vi "Main.vi"(11 "Module Admin":refnum<class "Delacor_lib_QMH_Module Admin.lvclass">) -> ()   [LabVIEW 2019, in "UI.lvlib"]
doc: "This template is based off of the Queued Message Handler design pattern and the Queued Message Handler project template that ships with LabVIEW.\n\nThe main difference is that the queue is private to this module and communication between modules is performed via Broadcast and Request events.\n\nRequest events are wrapped in public API methods and are handled in the Event Handling Loop (EHL) of this VI. Any module can register for Broadcast events sent by this module. The EHL generates messages based on user interface actions.\n\nThe Message Handling Loop (MHL) processes messages generated by the EHL, or by other messages. The messages are string values, so new messages can be added easily to the Message Cases case structure in the MHL. Each message cluster can also provide an optional value for Message Data, which is a variant that can be converted to whatever message-specific data is required.\n_____\nBased on Delacor QMH Project Template 5.0.0.82."
uses:
  UI.lvlib
  <vilib>/Delacor/Delacor QMH/Libraries/Module Admin_class/Delacor_lib_QMH_Module Admin.lvclass
  Module Data--cluster.ctl
  Stop Argument--cluster.ctl
  <vilib>/Delacor/Delacor QMH/Libraries/Message Queue_class/Delacor_lib_QMH_Message Queue.lvclass/Delacor_lib_QMH_Message Queue.ctl
  <vilib>/Delacor/Delacor QMH/Libraries/Module Admin_class/Delacor_lib_QMH_Module Admin.lvclass/Delacor_lib_QMH_Module Admin.ctl
  <vilib>/Delacor/Delacor QMH/Libraries/Message Queue_class/Delacor_lib_QMH_Enqueue Message (Single).vi
  <vilib>/Delacor/Delacor QMH/Libraries/Module Admin_class/Delacor_lib_QMH_Get External Launch.vi
  <vilib>/Utility/error.llb/Error Cluster From Error Code.vi
  <vilib>/ErrorRing/Error Ring.xnode
  <vilib>/Delacor/Delacor QMH/Libraries/Message Queue_class/Delacor_lib_QMH_Message Queue.lvclass
  Analisis/Analisis.lvlib
  Mensajes/Mensajes.lvlib
  Configuracion/Configuracion.lvlib
  Adquisicion_Helper_Loop/Adquisicion_Helper_Loop.lvlib
  Save DB_SQLite/Save DB_SQLite.lvlib
panel:
  out "error out":errorcluster
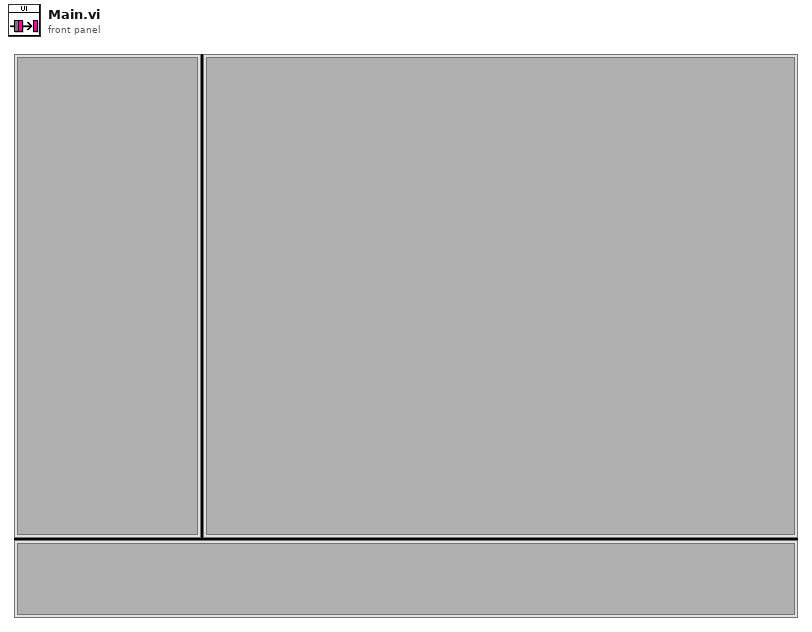
[diagram p1: front panel]
types:
  T1 = typedef "UI.lvlib/Request Events--cluster.ctl" = cluster{"Stop Module":refnum<user-event>, "Show Panel":refnum<user-event>, "Hide Panel":refnum<user-event>, "Get Module Execution Status":refnum<user-event>, "Show Diagram":refnum<user-event>}
  T2 = typedef "Configuracion.lvlib/Broadcast Events--cluster.ctl" = cluster{"Module Did Init":refnum<user-event>, "Status Updated":refnum<user-event>, "Error Reported":refnum<user-event>, "Module Did Stop":refnum<user-event>, "Update Module Execution Status":refnum<user-event>}
  T3 = typedef "Save DB_SQLite.lvlib/Broadcast Events--cluster.ctl" = cluster{"Module Did Init":refnum<user-event>, "Status Updated":refnum<user-event>, "Error Reported":refnum<user-event>, "Module Did Stop":refnum<user-event>, "Update Module Execution Status":refnum<user-event>}
  T4 = typedef "Mensajes.lvlib/Broadcast Events--cluster.ctl" = cluster{"Module Did Init":refnum<user-event>, "Status Updated":refnum<user-event>, "Error Reported":refnum<user-event>, "Module Did Stop":refnum<user-event>, "Update Module Execution Status":refnum<user-event>}
  T5 = typedef "Adquisicion_Helper_Loop.lvlib/Broadcast Events--cluster.ctl" = cluster{"Module Did Init":refnum<user-event>, "Status Updated":refnum<user-event>, "Error Reported":refnum<user-event>, "Module Did Stop":refnum<user-event>, "Update Module Execution Status":refnum<user-event>}
  T6 = typedef "Analisis.lvlib/Broadcast Events--cluster.ctl" = cluster{"Module Did Init":refnum<user-event>, "Status Updated":refnum<user-event>, "Error Reported":refnum<user-event>, "Module Did Stop":refnum<user-event>, "Update Module Execution Status":refnum<user-event>}
  T7 = typedef "UI.lvlib/Module Data--cluster.ctl" = cluster{"Status":string}
  T8 = enum32{"invalid lock state", "Not Locked", "Locked (No Password)", "Password-protected"}
  T9 = typedef "UI.lvlib/Stop Argument--cluster.ctl" = cluster{"Origin":string, "Exit via Stop Module Req?":bool, "Wait for Module to stop?":bool}
  T10 = enum32{"Invalid", "Standard", "Closed", "Hidden", "Minimized", "Maximized"}
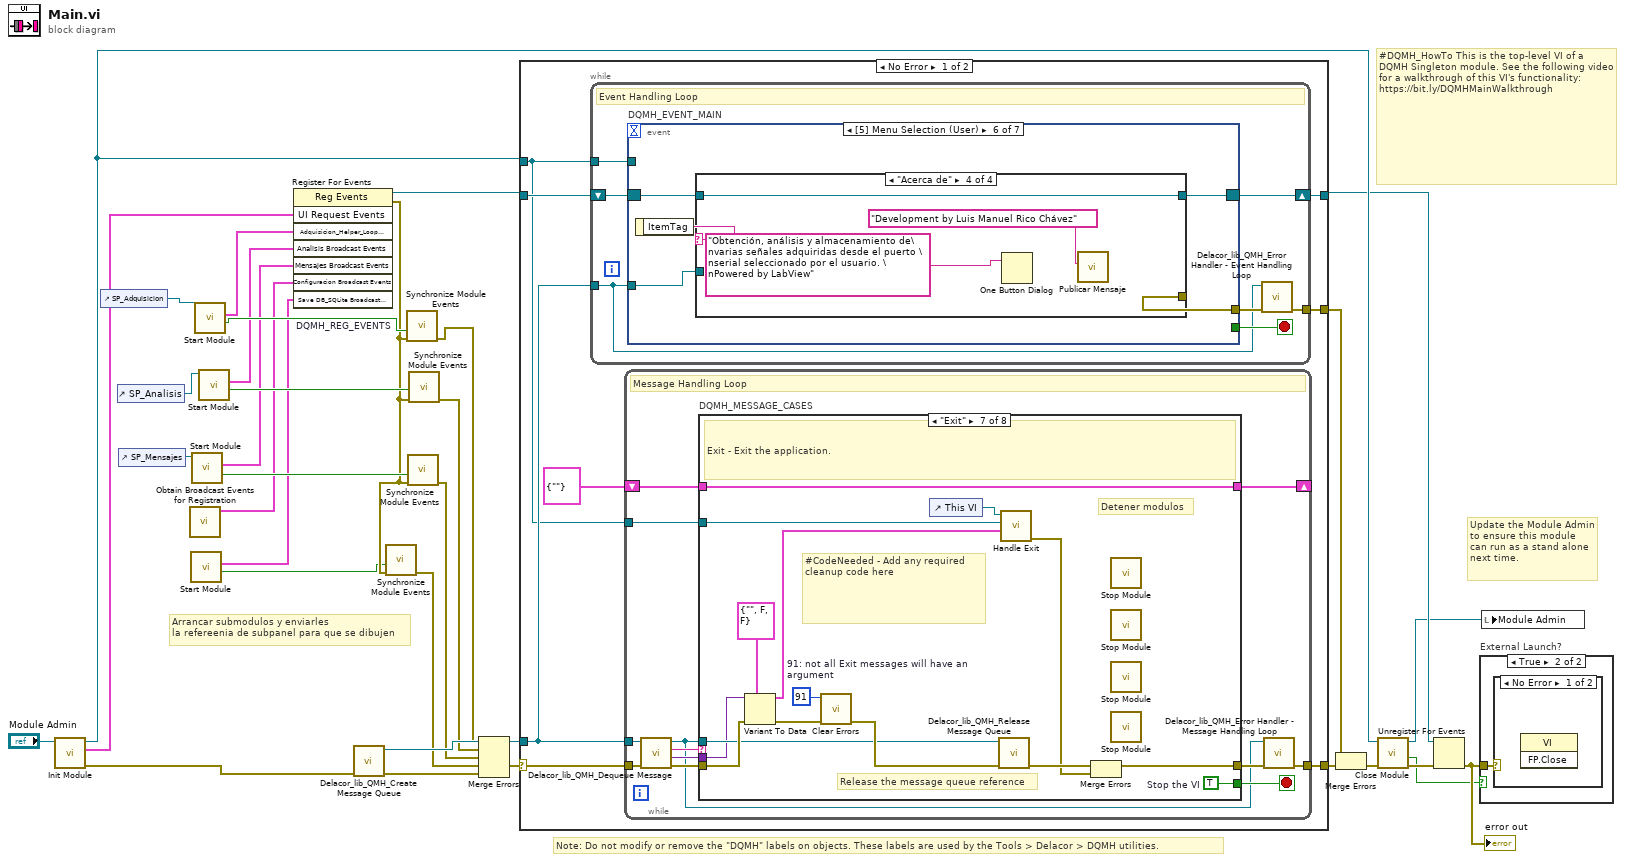
[diagram p0: block diagram]
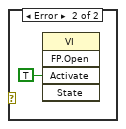
[diagram p3: hidden frame]
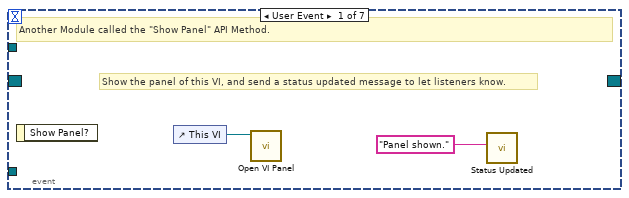
[diagram p4: hidden frame]
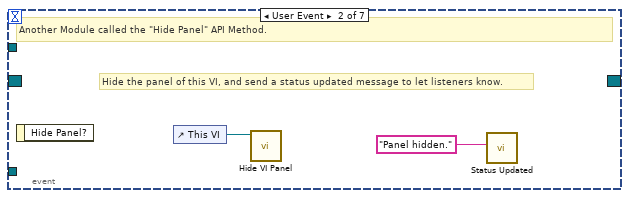
[diagram p5: hidden frame]
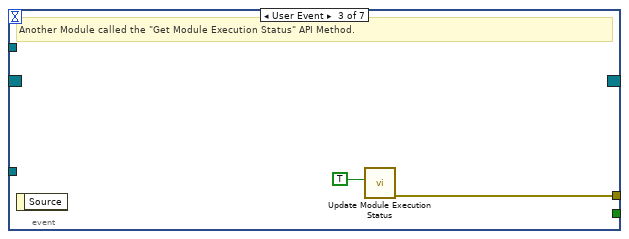
[diagram p6: hidden frame]
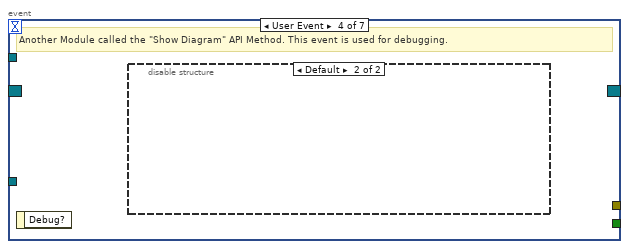
[diagram p7: hidden frame]
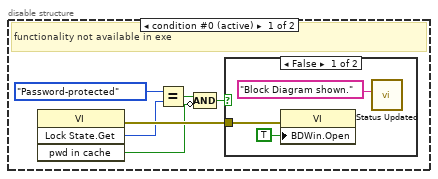
[diagram p8: hidden frame]
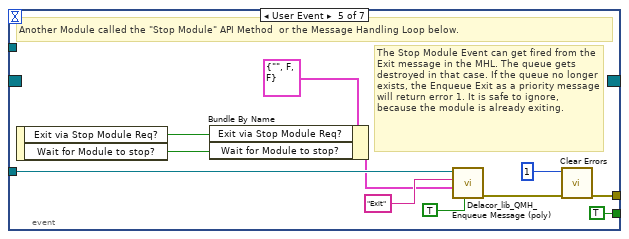
[diagram p10: hidden frame]
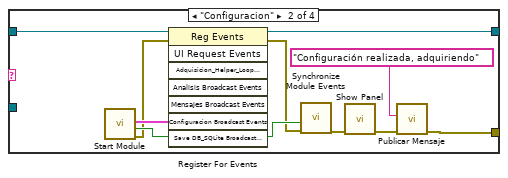
[diagram p12: hidden frame]
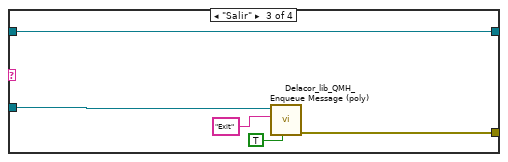
[diagram p13: hidden frame]
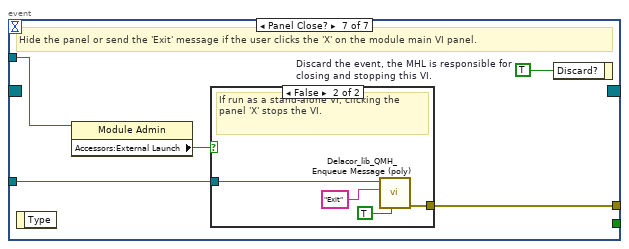
[diagram p14: hidden frame]
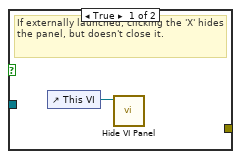
[diagram p15: hidden frame]
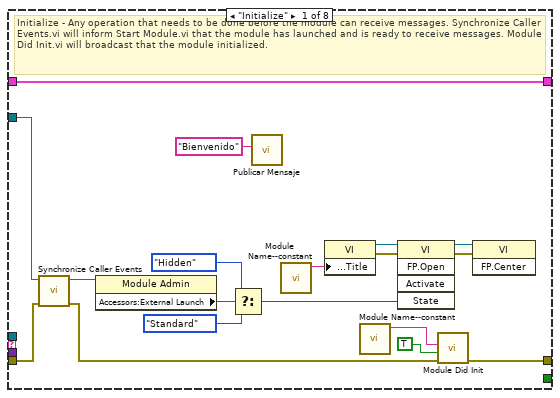
[diagram p16: hidden frame]
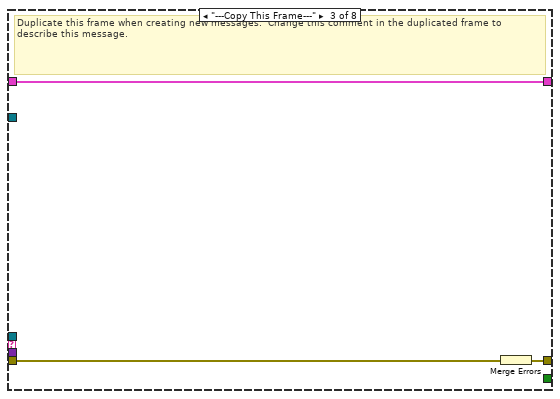
[diagram p18: hidden frame]
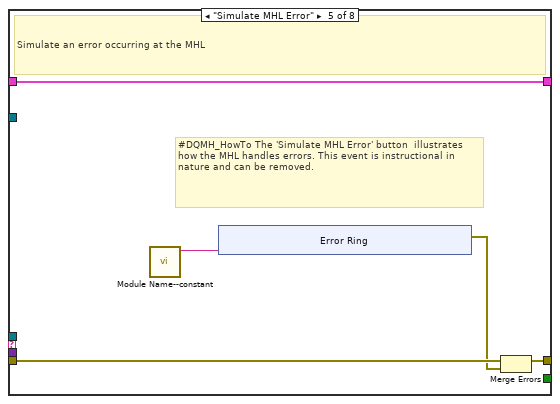
[diagram p20: hidden frame]
diagram:
  # "Arrancar submodulos y enviarles\nla refereenia de subpanel para que se dibujen"
  # "#DQMH_HowTo This is the top-level VI of a DQMH Singleton module. See the following video for a walkthrough of this VI's functionality: https://bit.ly/DQMHMainWalkthrough"
  # "Note: Do not modify or remove the \"DQMH\" labels on objects. These labels are used by the Tools > Delacor > DQMH utilities."
  # "Update the Module Admin to ensure this module can run as a stand alone next time."
  n1 = call "Init Module.vi"("Singleton Module Admin in"="Module Admin") -> ("error out"=w32:errorcluster, "UI Request Events"=w23:T1, "Singleton Module Admin out"=w26:refnum<class "Delacor_lib_QMH_Module Admin.lvclass">)  [unwired: 8 in]
  n2 = control-ref of="SP_Adquisicion"() -> (w9:refnum<vi>)
  n3 = control-ref of="SP_Analisis"() -> (w8:refnum<vi>)
  n4 = control-ref of="SP_Mensajes"() -> (w7:refnum<vi>)
  n5 = call "Obtain Broadcast Events for Registration.vi"() -> ("Configuracion Broadcast Events"=w6:T2)  [unwired: 9 in, 2 out]
  n6 = call "Start Module.vi"() -> ("Wait for Event Sync?"=w1:bool, "Save DB_SQLite Broadcast Events"=w5:T3)  [unwired: 8 in, 2 out]
  n7 = call "Start Module.vi"("SP_Mensajes"=w7) -> ("Wait for Event Sync?"=w16:bool, "Mensajes Broadcast Events"=w10:T4)  [unwired: 7 in, 2 out]
  n8 = call "Start Module.vi"("Sub Panel"=w9) -> ("Wait for Event Sync?"=w18:bool, "Adquisicion_Helper_Loop Broadcast Events"=w12:T5)  [unwired: 7 in, 2 out]
  n9 = call "Start Module.vi"("SP_Analisis"=w8) -> ("Wait for Event Sync?"=w17:bool, "Analisis Broadcast Events"=w11:T6)  [unwired: 7 in, 2 out]
  n10 = register-events "DQMH_REG_EVENTS"(w23, w12, w11, w10, w6, w5) -> (reference out=w24:refnum<event-registration>, error out=w2:errorcluster)  [unwired: 2 in]
  n11 = call <vilib>:"Delacor_lib_QMH_Create Message Queue.vi"("error in (no error)"=w32) -> ("error out"=w4:errorcluster, "Message Queue"=w22:refnum<class "Delacor_lib_QMH_Message Queue.lvclass">)  [unwired: 9 in]
  n12 = call "Synchronize Module Events.vi"("error in (no error)"=w2, "Wait for Event Sync?"=w1) -> ("error out"=w3:errorcluster)  [unwired: 9 in]
  n13 = call "Synchronize Module Events.vi"("error in (no error)"=w2, "Wait for Event Sync?"=w18) -> ("error out"=w13:errorcluster)  [unwired: 9 in]
  n14 = call "Synchronize Module Events.vi"("error in (no error)"=w2, "Wait for Event Sync?"=w16) -> ("error out"=w15:errorcluster)  [unwired: 9 in]
  n15 = call "Synchronize Module Events.vi"("error in (no error)"=w2, "Wait for Event Sync?"=w17) -> ("error out"=w14:errorcluster)  [unwired: 9 in]
  n16 = Merge Errors(w13, w14, w15, w3, w4) -> (w27:errorcluster)
  n17 = case shown="No Error" w27 {
    selector: w27 -> [w39 w206]
    tunnel: [w41 w205] -> w33
    tunnel: [w38 w211] -> w25
    tunnel: w24 -> [w36 w211]
    tunnel: w22 -> [w35 w204]
    tunnel: [w40 _] -> w30
    tunnel: w26 -> [w34 w207]
    frame No Error {
      n18 = while {
        tunnel: w35 -> [w42]
        shift-right: [w45] -> w38
        shift-left: w36 -> [w46]
        tunnel: [w47] -> w40
        tunnel: w34 -> [w43]
        stop <- w44 stop-if-true
        # "Event Handling Loop"
        n19 = event "DQMH_EVENT_MAIN" shown="[5] Menu Selection (User)" {
          selector: w46 -> [_ _ _ _ _ w77 _]
          dyn-events: [_ _ _ _ _ w76 _] -> w45
          timeout: _ -> [_ _ _ _ _ _ _]
          tunnel: [_ _ _ _ TRUE ("Discard?") _ _] -> w44
          tunnel: w42 -> [_ _ _ _ w70 w78 w101]
          tunnel: [_ _ w54 _ w73 w75 w103] -> w48
          tunnel: w43 -> [_ _ _ _ _ _ w100]
          event User Event {
            # "Show the panel of this VI, and send a status updated message to let listeners know."
            # "Another Module called the \"Show Panel\" API Method."
            n20 = event-data() -> ()  [unwired: 1 in, 1 out]
            n21 = control-ref of="This VI"() -> (w50:refnum<vi>)
            n22 = call "Open VI Panel.vi"("VI"=w50) -> ()  [unwired: 10 in, 1 out]
            n23 = call "Status Updated.vi"("Status"="Panel shown." ("format string")) -> ()  [unwired: 10 in, 1 out]
          }
          event User Event {
            # "Hide the panel of this VI, and send a status updated message to let listeners know."
            # "Another Module called the \"Hide Panel\" API Method."
            n24 = event-data() -> ()  [unwired: 1 in, 1 out]
            n25 = control-ref of="This VI"() -> (w52:refnum<vi>)
            n26 = call "Hide VI Panel.vi"("VI"=w52) -> ()  [unwired: 10 in, 1 out]
            n27 = call "Status Updated.vi"("Status"="Panel hidden." ("format string")) -> ()  [unwired: 10 in, 1 out]
          }
          event User Event {
            # "Another Module called the \"Get Module Execution Status\" API Method."
            n28 = event-data() -> ()  [unwired: 1 in, 1 out]
            n29 = call "Update Module Execution Status.vi"("Running?"=TRUE) -> ("error out"=w54:errorcluster)  [unwired: 10 in]
          }
          event User Event {
            # "Another Module called the \"Show Diagram\" API Method. This event is used for debugging."
            n30 = event-data() -> ()  [unwired: 1 in, 1 out]
            n31 = disable-structure shown="Default" {
              frame condition #0 (active) {
                # "functionality not available in exe"
                n32 = invoke class="VI" method="Lock State.Get"() -> (error out=w60:errorcluster, "Get Lock State"=w59:T8, "pwd in cache"=w56:bool)  [unwired: 4 in, 1 out]
                n33 = Equal?(x=T8."Password-protected", y=w59) -> (x = y?=w57:bool)
                n34 = Compound Arithmetic op=AND(w57, invert w56) -> (w55:bool)
                n35 = case shown="False" w55 {
                  tunnel: w60 -> [w63 _]
                  frame False {
                    n36 = property class="VI"(error in=w63, "BDWin.Open"=TRUE ("Block Diagram Window:Open")) -> ()  [unwired: 1 in, 2 out]
                    n37 = call "Status Updated.vi"("Status"="Block Diagram shown." ("format string")) -> ()  [unwired: 10 in, 1 out]
                  }
                  frame True {
                    # "Password-protected VI, and the password is not in the cache. Do not show the diagram."
                  }
                }
              }
              frame condition #1 {
              }
            }
          }
          event User Event {
            # "The Stop Module Event can get fired from the Exit message in the MHL. The queue gets destroyed in that case. If the queue no longer exists, the Enqueue Exit as a priority message will return error 1. It is safe to ignore, because the module is already exiting."
            # "Another Module called the \"Stop Module\" API Method  or the Message Handling Loop below."
            n38 = event-data() -> ("Exit via Stop Module Req?"=w66:bool, "Wait for Module to stop?"=w65:bool)  [unwired: 1 in]
            n39 = Bundle By Name(cluster=T9 {"Origin"="", "Exit via Stop Module Req?"=FALSE, "Wait for Module to stop?"=FALSE} ("Stop Argument"), "Exit via Stop Module Req?"=w66, "Wait for Module to stop?"=w65) -> (w64:T9)
            n40 = call-poly <vilib>:"Delacor_lib_QMH_Enqueue Message (poly).vi"("Priority Message? (F)"=TRUE, "Message Data"=w64, "Message"="Exit", "Message Queue in"=w70) -> ("error out"=w74:errorcluster)  [unwired: 6 in, 1 out]
            n41 = call <vilib>:"Clear Errors.vi"("error in (no error)"=w74, "specific error code to clear (0: all)"=1) -> ("error out"=w73:errorcluster)  [unwired: 4 in, 1 out]
          }
          event Menu Selection (User) {
            n42 = event-data() -> ("ItemTag"=w79:string)  [unwired: 1 in]
            n43 = case shown="\"Acerca de\"" w79 {
              tunnel: w78 -> [_ _ w93 _]
              tunnel: w77 -> [w80 w90 w92 w98]
              tunnel: [w80 w89 w92 w98] -> w76
              tunnel: [_ w81 w91 _] -> w75
              frame "False", Default {
              }
              frame "Configuracion" {
                n44 = call "Start Module.vi"() -> ("error out"=w86:errorcluster, "Wait for Event Sync?"=w87:bool, "Configuracion Broadcast Events"=w88:T2)  [unwired: 8 in, 1 out]
                n45 = register-events(reference=w90, error in=w86, w88) -> (reference out=w89:refnum<event-registration>, error out=w85:errorcluster)  [unwired: 5 in]
                n46 = call "Synchronize Module Events.vi"("error in (no error)"=w85, "Wait for Event Sync?"=w87) -> ("error out"=w84:errorcluster)  [unwired: 9 in]
                n47 = call "Show Panel.vi"("error in (no error)"=w84) -> ("error out"=w82:errorcluster)  [unwired: 10 in]
                n48 = call "Publicar Mensaje.vi"("error in (no error)"=w82, "Mensaje"="Configuración realizada, adquiriendo") -> ("error out"=w81:errorcluster)  [unwired: 9 in]
              }
              frame "Salir" {
                n49 = call-poly <vilib>:"Delacor_lib_QMH_Enqueue Message (poly).vi"("Priority Message? (F)"=TRUE, "Message"="Exit", "Message Queue in"=w93) -> ("error out"=w91:errorcluster)  [unwired: 7 in, 1 out]
              }
              frame "Acerca de" {
                n50 = One Button Dialog(message="Obtención, análisis y almacenamiento de\nvarias señales adquiridas desde el puerto \nserial seleccionado por el usuario. \nPowered by LabView") -> ()  [unwired: 1 in, 1 out]
                n51 = call "Publicar Mensaje.vi"("Mensaje"="Development by Luis Manuel Rico Chávez") -> ()  [unwired: 10 in, 1 out]
              }
            }
          }
          event Panel Close? {
            w102 = TRUE  # Discard the event, the MHL is responsible for closing and stopping this VI.
            # "Hide the panel or send the 'Exit' message if the user clicks the 'X' on the module main VI panel."
            n52 = event-data() -> ()  [unwired: 1 in, 1 out]
            n53 = property class="Module Admin"(reference=w100) -> ("Accessors:External Launch"=w99:bool)  [unwired: 1 in, 2 out]
            n54 = case shown="False" w99 {
              tunnel: w101 -> [_ w107]
              tunnel: [_ w108] -> w103
              frame True {
                # "If externally launched, clicking the 'X' hides the panel, but doesn't close it."
                n55 = control-ref of="This VI"() -> (w104:refnum<vi>)
                n56 = call "Hide VI Panel.vi"("VI"=w104) -> ()  [unwired: 10 in, 1 out]
              }
              frame False {
                # "If run as a stand-alone VI, clicking the panel 'X' stops the VI."
                n57 = call-poly <vilib>:"Delacor_lib_QMH_Enqueue Message (poly).vi"("Priority Message? (F)"=TRUE, "Message"="Exit", "Message Queue in"=w107) -> ("error out"=w108:errorcluster)  [unwired: 7 in, 1 out]
              }
            }
            n58 = event-data("Discard?"=w102) -> ()  [unwired: 1 in, 1 out]
          }
        }
        n59 = call-dynamic "Delacor_lib_QMH_Error Handler - Event Handling Loop.vi"("error in (no error)"=w48, "Message Queue in"=w42) -> ("dup error in"=w47:errorcluster)  [unwired: 8 in, 1 out]
      }
      n60 = while {
        tunnel: w35 -> [w111]
        shift-right: [w115] -> _
        shift-left: T7 {"Status"=""} ("Data Cluster") -> [w116]
        tunnel: w39 -> [w119]
        tunnel: [w117] -> w41
        tunnel: w34 -> [w109]
        stop <- w114 stop-if-true
        # "Message Handling Loop"
        n61 = call-dynamic "Delacor_lib_QMH_Dequeue Message.vi"("error in (no error)"=w119, "Message Queue in"=w111) -> ("error out"=w118:errorcluster, "Message Data"=w112:variant, "Message"=w113:string, "Message Queue out"=w110:refnum<class "Delacor_lib_QMH_Message Queue.lvclass">)  [unwired: 6 in]
        n62 = case "DQMH_MESSAGE_CASES" shown="\"Exit\"" w113 {
          selector: w113 -> [_ _ _ _ _ _ _ w191]
          tunnel: w110 -> [_ _ _ _ _ w161 w183 _]
          tunnel: w118 -> [w136 w140 w143 w145 w150 w168 w189 w193]
          tunnel: [w134 w140 w142 w145 w149 w164 w186 w194] -> w120
          tunnel: w116 -> [w125 w139 w141 w144 w147 w163 w182 w192]
          tunnel: [w125 w139 w141 w144 w147 w163 w182 w192] -> w115
          tunnel: [_ _ _ _ _ _ w181 _] -> w114
          tunnel: w112 -> [_ _ _ _ _ w162 w180 _]
          tunnel: w109 -> [w126 _ _ _ _ w160 w175 _]
          frame "Initialize" {
            # "Initialize - Any operation that needs to be done before the module can receive messages. Synchronize Caller Events.vi will inform Start Module.vi that the module has launched and is ready to receive messages. Module Did Init.vi will broadcast that the module initialized."
            n63 = call "Synchronize Caller Events.vi"("error in (no error)"=w136, "Singleton Module Admin in"=w126) -> ("error out"=w135:errorcluster, "Singleton Module Admin out"=w122:refnum<class "Delacor_lib_QMH_Module Admin.lvclass">)  [unwired: 8 in]
            n64 = property class="Module Admin"(reference=w122) -> ("Accessors:External Launch"=w130:bool)  [unwired: 1 in, 2 out]
            n65 = Select(t=T10."Hidden" ("State"), s=w130, f=T10."Standard" ("State")) -> (s? t:f=w127:T10)
            n66 = call "Publicar Mensaje.vi"("Mensaje"="Bienvenido") -> ()  [unwired: 10 in, 1 out]
            n67 = call "Module Name--constant.vi"() -> ("Module Name"=w133:string)  [unwired: 11 in]
            n68 = property class="VI"("Front Panel.Title"=w133) -> (reference out=w132:refnum<vi>, error out=w138:errorcluster)  [unwired: 2 in]
            n69 = call "Module Name--constant.vi"() -> ("Module Name"=w123:string)  [unwired: 11 in]
            n70 = invoke class="VI" method="FP.Open"(reference=w132, error in=w138, "State"=w127) -> (reference out=w131:refnum<vi>, error out=w137:errorcluster)  [unwired: 2 in, 3 out]
            n71 = call "Module Did Init.vi"("error in (no error)"=w135, "Initialized?"=TRUE, "Origin"=w123) -> ("error out"=w134:errorcluster)  [unwired: 8 in]
            n72 = invoke class="VI" method="FP.Center"(reference=w131, error in=w137) -> ()  [unwired: 1 in, 3 out]
          }
          frame "--- Module Specific ---" {
            # "Separator -- The following cases handle messages specific to this Module."
          }
          frame "---Copy This Frame---" {
            # "Duplicate this frame when creating new messages.  Change this comment in the duplicated frame to describe this message."
            n73 = Merge Errors(w143) -> (w142:errorcluster)
          }
          frame "--- Exit and Error Handling---" {
            # "Separator - The following cases handle errors and exit messages."
          }
          frame "Simulate MHL Error" {
            # "#DQMH_HowTo The 'Simulate MHL Error' button  illustrates how the MHL handles errors. This event is instructional in nature and can be removed."
            # "Simulate an error occurring at the MHL"
            n74 = call "Module Name--constant.vi"() -> ("Module Name"=w146:string)  [unwired: 11 in]
            n75 = xnode "Error Ring"("parameter 0"=w146) -> ("error out"=w148:errorcluster)
            n76 = Merge Errors(w150, w148) -> (w149:errorcluster)
          }
          frame "Error" {
            # "#CodeRecommended - If you ever change the name of this \"Error\" message, you'll need to update the name in the Check Loop Error.vi as well."
            # "#CodeRecommended - If the module is running in standalone mode (External Launch = FALSE), this code will pop up an error dialog and call the 'Exit' message if an error occurs. Add more fine-grained error handling here."
            # "Error - Check the error message data and respond accordingly. This message is sent by the \"Error Handler\" VIs at the end of each loop in this application."
            n77 = property class="Module Admin"(reference=w160) -> ("Accessors:External Launch"=w159:bool)  [unwired: 1 in, 2 out]
            n78 = Variant To Data(error in=w168, type=errorcluster {"status"=FALSE, "code"=0, "source"=""} ("error constant"), Variant=w162) -> (data=w169:errorcluster, error out=w166:errorcluster)
            n79 = call "Module Name--constant.vi"() -> ("Module Name"=w158:string)  [unwired: 11 in]
            n80 = call "Error Reported.vi"("Additional Information"=w158, "Error"=w169) -> ()  [unwired: 9 in, 1 out]
            n81 = case shown="False" w159 {
              tunnel: [w174 _] -> w165
              tunnel: w161 -> [w172 _]
              tunnel: w169 -> [w173 _]
              frame False {
                # "If the module is running standalone, then pop up an error dialog and call the \"Exit\" message."
                n82 = call <vilib>:"Simple Error Handler.vi"("error in (no error)"=w173) -> ()  [unwired: 4 in, 5 out]
                n83 = call-poly <vilib>:"Delacor_lib_QMH_Enqueue Message (poly).vi"("Priority Message? (F)"=TRUE, "Message"="Exit", "Message Queue in"=w172) -> ("error out"=w174:errorcluster)  [unwired: 7 in, 1 out]
              }
              frame True {
                # "If the module was launched externally, calling the Error Reported broadcast VI is the only action performed by the \"Error\" message. The module's caller can then process the error appropriately."
              }
            }
            n84 = Merge Errors(w166, w165) -> (w164:errorcluster)
            n85 = local write "error out"(w164) -> ()
          }
          frame "Exit" {
            w179 = 91  # 91: not all Exit messages will have an argument
            w181 = TRUE  # Stop the VI
            # "Detener modulos"
            # "Release the message queue reference"
            # "#CodeNeeded - Add any required cleanup code here"
            # "Exit - Exit the application."
            n86 = Variant To Data(error in=w189, type=T9 {"Origin"="", "Exit via Stop Module Req?"=FALSE, "Wait for Module to stop?"=FALSE} ("Stop Argument"), Variant=w180) -> (data=w177:T9, error out=w185:errorcluster)
            n87 = call <vilib>:"Clear Errors.vi"("error in (no error)"=w185, "specific error code to clear (0: all)"=w179) -> ("error out"=w188:errorcluster)  [unwired: 4 in, 1 out]
            n88 = control-ref of="This VI"() -> (w176:refnum<vi>)
            n89 = call-dynamic "Delacor_lib_QMH_Release Message Queue.vi"("error in (no error)"=w188, "Message Queue"=w183) -> ("error out"=w187:errorcluster)  [unwired: 9 in]
            n90 = call "Handle Exit.vi"("Stop Argument"=w177, "Admin in"=w175, "VI reference"=w176) -> ("error out"=w184:errorcluster)  [unwired: 7 in, 1 out]
            n91 = Merge Errors(w187, w184) -> (w186:errorcluster)
            n92 = call "Stop Module.vi"() -> ()  [unwired: 11 in, 1 out]
            n93 = call "Stop Module.vi"() -> ()  [unwired: 11 in, 1 out]
            n94 = call "Stop Module.vi"() -> ()  [unwired: 11 in, 1 out]
            n95 = call "Stop Module.vi"() -> ()  [unwired: 11 in, 1 out]
          }
          frame Default {
            # "'Default' case only runs if there is a message that isn't defined in any of the other cases.  Output a programming error."
            n96 = call "Module Name--constant.vi"() -> ("Module Name"=w190:string)  [unwired: 11 in]
            n97 = xnode "Error Ring"("parameter 0"=w191, "parameter 1"=w190) -> ("error out"=w195:errorcluster)
            n98 = Merge Errors(w193, w195) -> (w194:errorcluster)
          }
        }
        n99 = call-dynamic "Delacor_lib_QMH_Error Handler - Message Handling Loop.vi"("error in (no error)"=w120, "Message Queue in"=w110) -> ("dup error in"=w117:errorcluster)  [unwired: 8 in, 1 out]
      }
    }
    frame Error {
      # "Synchronize Caller Events.vi will inform Start Module.vi that the module has launched and will let the code calling Start Module.vi register for broadcasts and would permit the caller receive the broadcast that an error occurred at launch time."
      n100 = call-dynamic "Delacor_lib_QMH_Release Message Queue.vi"("error in (no error)"=w206, "Message Queue"=w204) -> ("error out"=w205:errorcluster)  [unwired: 9 in]
      n101 = call "Synchronize Caller Events.vi"("Singleton Module Admin in"=w207) -> ("error out"=w212:errorcluster)  [unwired: 9 in, 1 out]
      n102 = call "Module Name--constant.vi"() -> ("Module Name"=w210:string)  [unwired: 11 in]
      n103 = Format Into String(format string="An error occurred during initialization. %s is no longer running.", w210) -> (resulting string=w208:string)  [unwired: 2 in, 1 out]
      n104 = Merge Errors(w205, w212) -> (w213:errorcluster)
      n105 = call "Error Reported.vi"("Additional Information"=w208, "Error"=w213) -> ()  [unwired: 9 in, 1 out]
    }
  }
  n106 = Merge Errors(w30, w33) -> (w29:errorcluster)
  n107 = call "Close Module.vi"("error in (no error)"=w29, "Module Admin in"=w26) -> ("error out"=w31:errorcluster, "External Launch"=w19:bool, "Module Admin out"=w20:refnum<class "Delacor_lib_QMH_Module Admin.lvclass">)  [unwired: 7 in]
  n108 = Unregister For Events(event registration refnum=w25, error in=w31) -> (error out=w28:errorcluster)
  "error out" <- w28
  n109 = case "External Launch?" shown="True" w19 {
    tunnel: w28 -> [_ w214]
    frame False {
    }
    frame True {
      n110 = case shown="No Error" w214 {
        frame No Error {
          n111 = invoke class="VI" method="FP.Close"() -> ()  [unwired: 3 in, 3 out]
        }
        frame Error {
          n112 = invoke class="VI" method="FP.Open"("Activate"=TRUE ("Activate?")) -> ()  [unwired: 4 in, 5 out]
        }
      }
    }
  }
  n113 = local write "Module Admin"(w20) -> ()
